vi "Counter global variable.vi"() -> ()   [LabVIEW 2021, in "Named Counters.lvlib"]
uses:
  Named Counters.lvlib
  Counter Cluster.ctl
panel:
  in  "Counters":T1[](array[typedef])
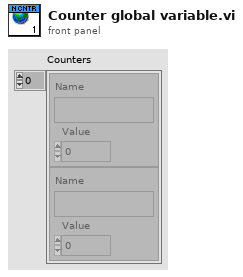
[diagram p1: front panel]
types:
  T1 = typedef "Named Counters.lvlib/Counter Cluster.ctl" = cluster{"Name":string, "Value":i32}
diagram:
